vi "Add Subpanel Tag.vi"(6 "subpanel UID":i32, 8 "error in":errorcluster, 9 "owning VI name":string, 10 "subpanel tag":string, 11 "state in":T1) -> (0 "error out":errorcluster, 3 "state out":T1)   [LabVIEW 2010, in "NI_SE_Config Front Panel Layout.lvlib"]
uses:
  NI_SE_Config Front Panel Layout.lvlib
  State.ctl
  VI Info.ctl
  VI Panel Layout/VI Panel Layout.lvclass
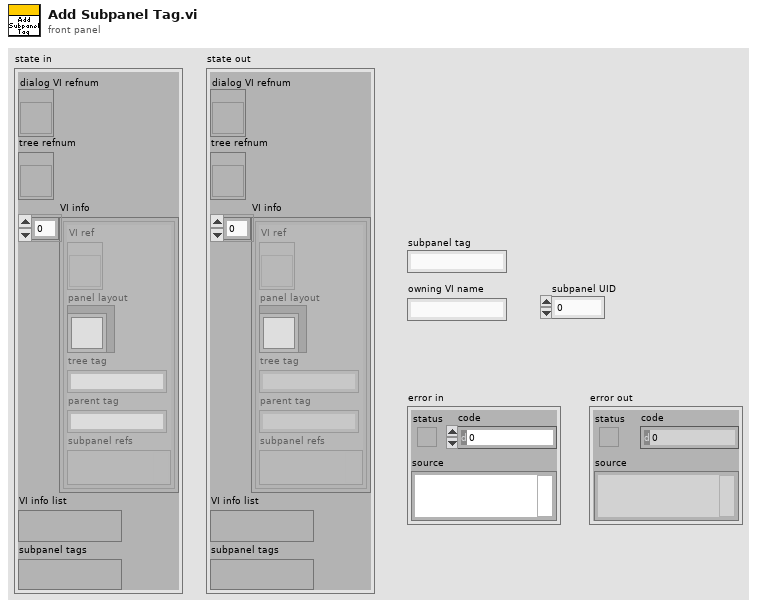
[diagram p1: front panel]
types:
  T1 = typedef "NI_SE_Config Front Panel Layout.lvlib/State.ctl" = cluster{"dialog VI refnum":refnum<vi>, "tree refnum":refnum<vi>, "VI info":T2[], "VI info list":variant, "subpanel tags":variant}
  T2 = typedef "NI_SE_Config Front Panel Layout.lvlib/VI Info.ctl" = cluster{"VI ref":refnum<vi>, "panel layout":refnum<class "VI Panel Layout.lvclass">, "tree tag":string, "parent tag":string, "subpanel refs":variant}
  T3 = cluster{"subpanel UID":i32, "owning VI name":string}
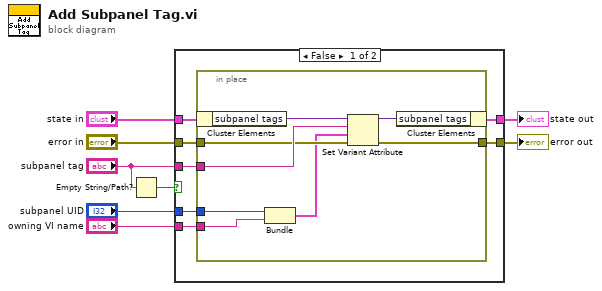
[diagram p0: block diagram]
diagram:
  n1 = Empty String/Path?(string/path="subpanel tag") -> (empty?=w2:bool)
  n2 = case shown="False" w2 {
    tunnel: "state in" -> [w15 w25]
    tunnel: "subpanel tag" -> [w14 _]
    tunnel: "error in" -> [w13 w24]
    tunnel: [w12 w24] -> w6
    tunnel: [w11 w25] -> w5
    tunnel: "owning VI name" -> [w10 _]
    tunnel: "subpanel UID" -> [w9 _]
    frame False {
      n3 = in-place {
        in-place-border: w14 -> [w21]
        in-place-border: w13 -> [w20]
        in-place-border: [w19] -> w12
        in-place-border: w10 -> [w17]
        in-place-border: w9 -> [w18]
        n4 = in-place-cluster #1(w15) -> ("subpanel tags"=w23:variant)
        n5 = Bundle("subpanel UID"=w18, "owning VI name"=w17) -> (w16:T3)  [unwired: 1 in]
        n6 = Set Variant Attribute(Variant=w23, name=w21, value=w16, error in=w20) -> (Variant out=w22:variant, error out=w19:errorcluster)  [unwired: 1 out]
        n7 = in-place-cluster #1("subpanel tags"=w22) -> (w11:T1)
      }
    }
    frame True {
    }
  }
  "state out" <- w5
  "error out" <- w6
